vi "LEDBegin.vi"   [LabVIEW 2023]
uses:
  <vilib>/Rock Robotics/SystemInterfaces/DIO/FPGA_DIOPWMChannel.ctl
types:
  T1 = typedef "FPGA_DIOPWMChannel.ctl" = enum8{"PWM 0", "PWM 1", "PWM 2", "PWM 3", "PWM 4", "PWM 5", "PWM 6", "PWM 7", "PWM 8", "PWM 9", "PWM MXP 0", "PWM MXP 1", "PWM MXP 2", "PWM MXP 3", "PWM MXP 4", "PWM MXP 5", "PWM MXP 6", "PWM MXP 7", "PWM MXP 8", "PWM MXP 9", "Invalid"}
  T2 = typedef "WPI_PWMDeviceRef.ctl" = cluster{"DeviceStatus":errorcluster, "PWM Channel":T1}
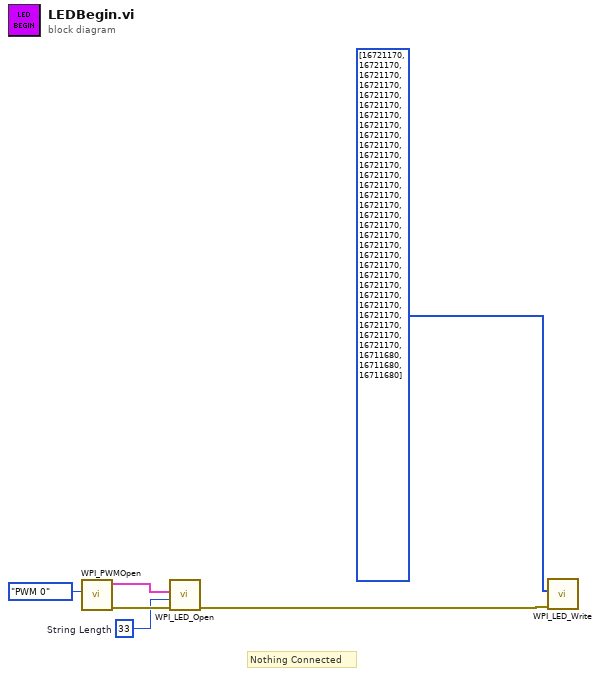
[diagram p0: block diagram]
diagram:
  w3 = u16 33  # String Length
  # "Nothing Connected"
  n1 = call <vilib>:"WPI_PWMOpen.vi"("PWM Channel"=FPGA_DIOPWMChannel."PWM 0") -> ("error out"=w4:errorcluster, "PWMDeviceRef"=w5:T2)  [unwired: 9 in]
  n2 = call <vilib>:"WPI_LED_Open.vi"("error in"=w4, "String Length"=w3, "PWMDeviceRef"=w5) -> ("error out"=w1:errorcluster)  [unwired: 8 in]
  n3 = call <vilib>:"WPI_LED_Write.vi"("error in"=w1, "Color Array"=u32[] [16721170, 16721170, 16721170, 16721170, 16721170, 16721170, 16721170, 16721170, 16721170, 16721170, 16721170, 16721170, 16721170, 16721170, 16721170, 16721170, 16721170, 16721170, 16721170, 16721170, 16721170, 16721170, 16721170, 16721170, 16721170, 16721170, 16721170, 16721170, 16721170, 16721170, 16711680, 16711680, 16711680]) -> ()  [unwired: 9 in, 1 out]
